vi "Panel Resized.vi"(6 "Sizing Refnums":T2, 8 "error in (no error)":errorcluster, 9 "Origin":cluster{"H":i16, "V":i16}, 10 "NewBnds":T1, 11 "Size Constraints":cluster{"min tab width":i32, "w/h":dbl}) -> (0 "error out":errorcluster)   [LabVIEW 2016]
uses:
  <vilib>/Utility/miscctls.llb/LVRectTypeDef.ctl
  <vilib>/Utility/miscctls.llb/LVRowAndColumnTypeDef.ctl
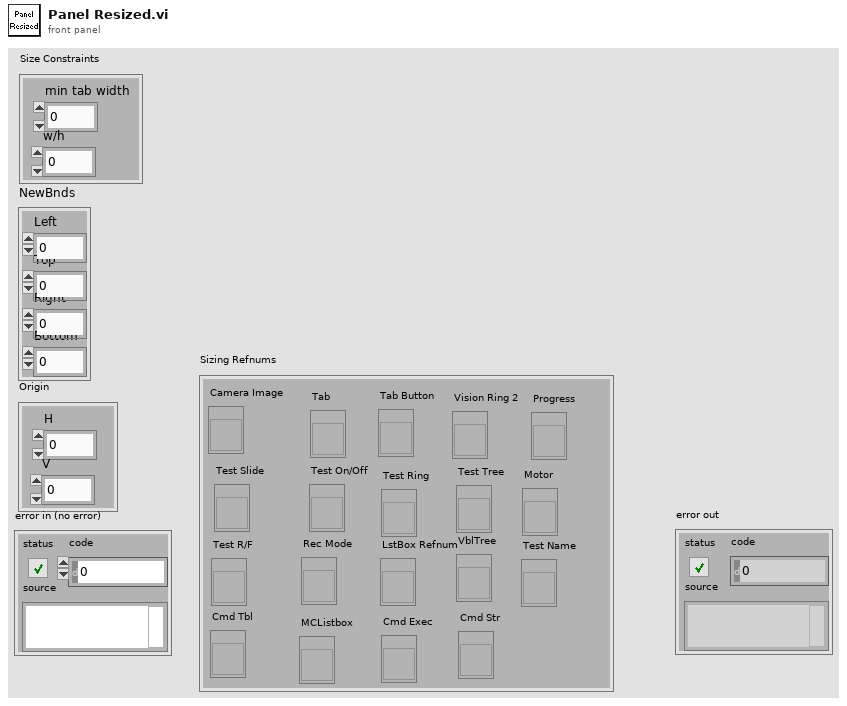
[diagram p1: front panel]
types:
  T1 = typedef "LVRectTypeDef.ctl" = cluster{"Left":i16, "Top":i16, "Right":i16, "Bottom":i16}
  T2 = cluster{"Camera Image":refnum<vi>, "Tab":refnum<vi>, "Tab Button":refnum<vi>, "Vision Ring 2":refnum<vi>, "Rec Mode":refnum<vi>, "Test Slide":refnum<vi>, "Test On/Off":refnum<vi>, "Test Ring":refnum<vi>, "Test R/F":refnum<vi>, "Test Name":refnum<vi>, "Motor":refnum<vi>, "Progress":refnum<vi>, "LstBox Refnum":refnum<vi>, "Test Tree":refnum<vi>, "VblTree":refnum<vi>, "Cmd Tbl":refnum<vi>, "MCListbox":refnum<vi>, "Cmd Exec":refnum<vi>, "Cmd Str":refnum<vi>}
  T3 = typedef "LVRowAndColumnTypeDef.ctl" = cluster{"Row":i32, "Column":i32}
  T4 = typedef "LVPositionTypeDef.ctl" = cluster{"Left":i32, "Top":i32}
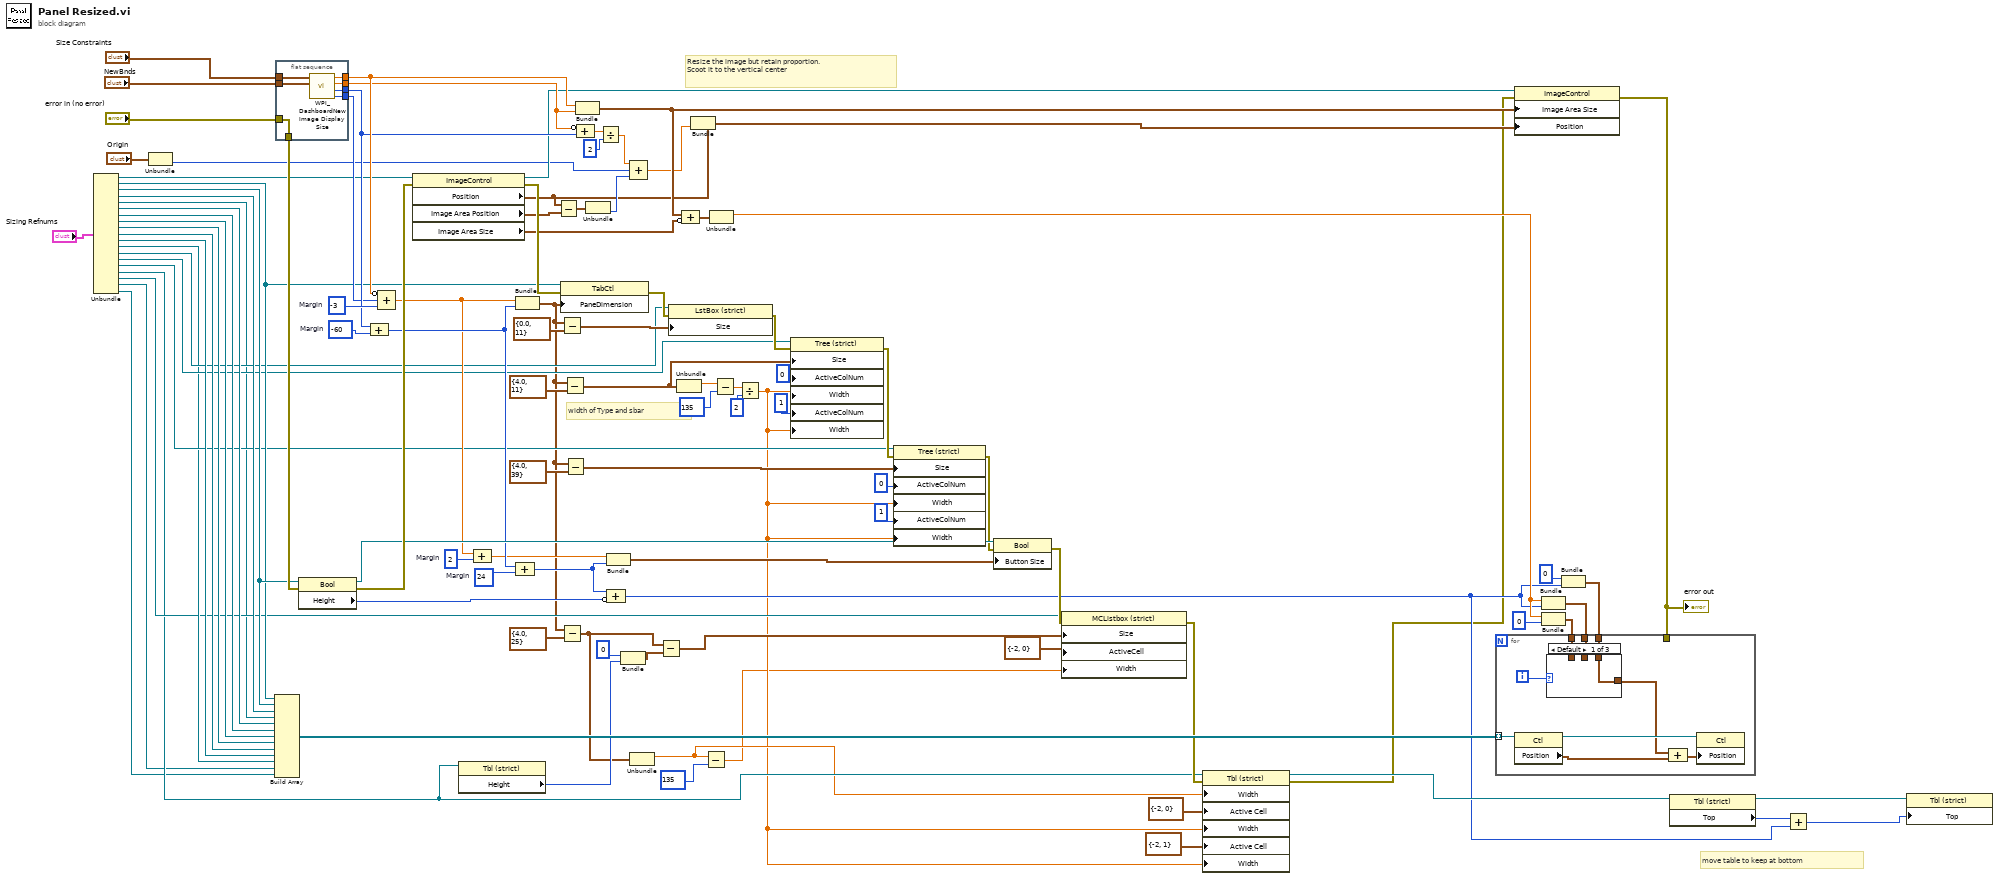
[diagram p0: block diagram]
diagram:
  w86 = 24  # Margin
  w84 = 2  # Margin
  w80 = -60  # Margin
  w90 = -3  # Margin
  # "move table to keep at bottom"
  # "width of Type and sbar"
  # "Resize the image but retain proportion.\nScoot it to the vertical center"
  n1 = Unbundle("Sizing Refnums") -> ("Camera Image"=w54:refnum<vi>, "Tab"=w55:refnum<vi>, "Tab Button"=w63:refnum<vi>, "Vision Ring 2"=w100:refnum<vi>, "Rec Mode"=w3:refnum<vi>, "Test Slide"=w101:refnum<vi>, "Test On/Off"=w102:refnum<vi>, "Test Ring"=w103:refnum<vi>, "Test R/F"=w104:refnum<vi>, "Test Name"=w35:refnum<vi>, "Motor"=w34:refnum<vi>, "Progress"=w28:refnum<vi>, "LstBox Refnum"=w29:refnum<vi>, "Test Tree"=w30:refnum<vi>, "VblTree"=w31:refnum<vi>, "Cmd Tbl"=w22:refnum<vi>, "MCListbox"=w23:refnum<vi>, "Cmd Exec"=w2:refnum<vi>, "Cmd Str"=w1:refnum<vi>)
  n2 = Unbundle("Origin") -> ("V"=w60:i16)  [unwired: 1 out]
  n3 = Build Array(w55, w63, w100, w3, w101, w102, w103, w104, w35, w34, w28, w2, w1) -> (w99:refnum<vi>[])
  n4 = flat-sequence {
    tunnel: "NewBnds" -> [w111]
    tunnel: "Size Constraints" -> [w110]
    tunnel: [w109] -> w79
    tunnel: [w108] -> w87
    tunnel: [w107] -> w88
    tunnel: [w106] -> w89
    tunnel: [w105] -> w98
    tunnel: "error in (no error)" -> [w105]
    frame #0 {
      n5 = call <vilib>:"WPI_DashboardNew Image Display Size.vi"("NewBnds"=w111, "Size Constraints"=w110) -> ("Window Width"=w109:i16, "Window Height"=w107:i16, "Height"=w108:dbl, "Width"=w106:dbl)  [unwired: 6 in]
    }
  }
  n6 = property class="Bool"(reference=w63, error in=w98) -> (reference out=w93:refnum<vi>, error out=w97:errorcluster, "Height"=w92:u32)
  n7 = Compound Arithmetic op=unknown(w88, w80) -> (w85:i32)
  n8 = Compound Arithmetic op=ADD(invert w89, w79, w90) -> (w83:dbl)
  n9 = property class="ImageControl"(reference=w54, error in=w97) -> (reference out=w72:refnum<vi>, error out=w96:errorcluster, "Position"=w71:T4, "Image Area Position"=w66:cluster{"Left":i32, "Top":i32}, "Image Area Size"=w77:cluster{"Width":u32, "Height":u32})
  n10 = property class="Tbl (strict)"(reference=w22) -> ("Height"=w21:u32)  [unwired: 1 in, 2 out]
  n11 = Compound Arithmetic op=ADD(w83, w84) -> (w82:dbl)
  n12 = Bundle(w83, w85) -> (w16:cluster{dbl, i32})  [unwired: 1 in]
  n13 = Compound Arithmetic op=ADD(w85, w86) -> (w91:i32)
  n14 = Subtract(x=w71, y=w66) -> (x-y=w73:T4)
  n15 = property class="TabCtl"(reference=w55, error in=w96, "PaneDimension"=w16) -> (error out=w53:errorcluster)  [unwired: 1 out]
  n16 = Subtract(x=w16, y=cluster{dbl, i32} {0.0, 11}) -> (x-y=w52:cluster{dbl, i32})
  n17 = Subtract(x=w16, y=cluster{dbl, i32} {4.0, 25}) -> (x-y=w18:cluster{dbl, i32})
  n18 = Subtract(x=w16, y=cluster{dbl, i32} {4.0, 11}) -> (x-y=w42:cluster{dbl, i32})
  n19 = Subtract(x=w16, y=cluster{dbl, i32} {4.0, 39}) -> (x-y=w48:cluster{dbl, i32})
  n20 = Bundle("Width"=w89, "Height"=w87) -> (w75:cluster{"Width":dbl, "Height":dbl})  [unwired: 1 in]
  n21 = Compound Arithmetic op=ADD(invert w87, w88) -> (w67:dbl)
  n22 = Unbundle(w73) -> ("Top"=w74:i32)  [unwired: 1 out]
  n23 = Divide(x=w67, y=2) -> (x/y=w69:dbl)
  n24 = Bundle(w82, w91) -> (w81:cluster{dbl, i32})  [unwired: 1 in]
  n25 = Compound Arithmetic op=ADD(w91, invert w92) -> (w12:u32)
  n26 = Bundle(0, "Height"=w21) -> (w19:cluster{i32, "Height":u32})  [unwired: 1 in]
  n27 = Compound Arithmetic op=ADD(w69, w60, w74) -> (w70:dbl)
  n28 = Unbundle(w18) -> (w7:dbl)  [unwired: 1 out]
  n29 = Subtract(x=w18, y=w19) -> (x-y=w17:cluster{dbl, u32})
  n30 = property class="LstBox (strict)"(reference=w29, error in=w53, "Size"=w52) -> (error out=w47:errorcluster)  [unwired: 1 out]
  n31 = Unbundle(w42) -> (w41:dbl)  [unwired: 1 out]
  n32 = Compound Arithmetic op=ADD(w75, invert w77) -> (w78:cluster{"Width":dbl, "Height":dbl})
  n33 = Bundle(cluster=w71, "Top"=w70) -> (w76:T4)  [unwired: 1 in]
  n34 = Subtract(x=w7, y=135) -> (x-y=w4:dbl)
  n35 = Unbundle(w78) -> ("Width"=w94:dbl)  [unwired: 1 out]
  n36 = Subtract(x=w41, y=135 ("Active Cell:Active Column Number")) -> (x-y=w37:dbl)
  n37 = Divide(x=w37, y=2 ("Active Cell:Active Column Number")) -> (x/y=w5:dbl)
  n38 = property class="Tree (strict)"(reference=w30, error in=w47, "Size"=w42, "ActiveColNum"=0 ("Active Cell:Active Column Number"), "Width"=w5, "ActiveColNum"=1 ("Active Cell:Active Column Number"), "Width"=w5) -> (error out=w46:errorcluster)  [unwired: 1 out]
  n39 = property class="Tree (strict)"(reference=w31, error in=w46, "Size"=w48, "ActiveColNum"=0 ("Active Cell:Active Column Number"), "Width"=w5, "ActiveColNum"=1 ("Active Cell:Active Column Number"), "Width"=w5) -> (error out=w45:errorcluster)  [unwired: 1 out]
  n40 = property class="Bool"(reference=w93, error in=w45, "Button Size"=w81) -> (error out=w27:errorcluster)  [unwired: 1 out]
  n41 = property class="MCListbox (strict)"(reference=w23, error in=w27, "Size"=w17, "ActiveCell"=T3 {"Row"=-2, "Column"=0} ("Active Cell:Active Cell"), "Width"=w4) -> (error out=w24:errorcluster)  [unwired: 1 out]
  n42 = property class="Tbl (strict)"(reference=w22, error in=w24, "Width"=w7, "Active Cell"=T3 {"Row"=-2, "Column"=0} ("Active Cell:Active Cell"), "Width"=w5, "Active Cell"=T3 {"Row"=-2, "Column"=1} ("Active Cell:Active Cell"), "Width"=w5) -> (reference out=w15:refnum<vi>, error out=w10:errorcluster)
  n43 = property class="ImageControl"(reference=w72, error in=w10, "Image Area Size"=w75, "Position"=w76) -> (error out=w59:errorcluster)  [unwired: 1 out]
  "error out" <- w59
  n44 = Bundle("Width"=w94, w12) -> (w65:cluster{"Width":dbl, u32})  [unwired: 1 in]
  n45 = Bundle("Width"=w94, 0) -> (w64:cluster{"Width":dbl, i32})  [unwired: 1 in]
  n46 = Bundle(0, w12) -> (w32:cluster{i32, u32})  [unwired: 1 in]
  n47 = for {
    tunnel: w99 -> [w120] mode=indexing
    tunnel: w65 -> [w114]
    tunnel: w64 -> [w115]
    tunnel: w59 -> [_]
    tunnel: w32 -> [w113]
    i -> [w116]
    n48 = property class="Ctl"(reference=w120) -> (reference out=w119:refnum<vi>, "Position"=w118:T4)  [unwired: 1 in, 1 out]
    n49 = case shown="Default" w116 {
      tunnel: w115 -> [_ w122 _]
      tunnel: w114 -> [_ _ w123]
      tunnel: w113 -> [w121 _ _]
      tunnel: [w121 w122 w123] -> w112
      frame Default {
      }
      frame 0, 1 {
      }
      frame 2, 3 {
      }
    }
    n50 = Compound Arithmetic op=ADD(w112, w118) -> (w117:cluster{dbl, u32})
    n51 = property class="Ctl"(reference=w119, "Position"=w117) -> ()  [unwired: 1 in, 2 out]
  }
  n52 = property class="Tbl (strict)"(reference=w15) -> (reference out=w14:refnum<vi>, "Top"=w13:i32)  [unwired: 1 in, 1 out]
  n53 = Add(x=w13, y=w12) -> (x+y=w11:u32)
  n54 = property class="Tbl (strict)"(reference=w14, "Top"=w11) -> ()  [unwired: 1 in, 2 out]
